vi "Area and Validity of a Triangle.vi"() -> ()   [LabVIEW 2011]
panel:
  out "Area of Triangle":dbl
  out "Valid Triangle?":bool
  in  "Side C (cm)":dbl=10.0
  in  "Side B (cm)":dbl=8.0
  in  "Side A (cm)":dbl=6.0
  # "Sides of a Triangle"
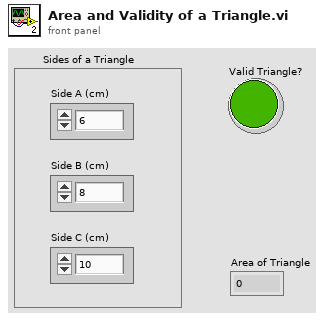
[diagram p1: front panel]
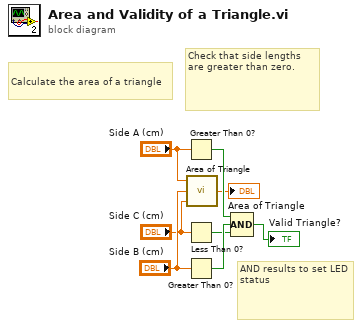
[diagram p0: block diagram]
diagram:
  # "AND results to set LED status"
  # "Check that side lengths are greater than zero."
  # "Calculate the area of a triangle"
  n1 = Greater Than 0?(x="Side A (cm)") -> (x > 0?=w8:bool)
  n2 = Less Than 0?(x="Side C (cm)") -> (x < 0?=w6:bool)
  n3 = Greater Than 0?(x="Side B (cm)") -> (x > 0?=w7:bool)
  n4 = call "Area of Triangle.vi"("Side C (cm)"="Side C (cm)", "Side B (cm)"="Side B (cm)", "Side A (cm)"="Side A (cm)") -> ("Area of Triangle (cm^2)"=→"Area of Triangle":dbl)
  n5 = Compound Arithmetic op=AND(w8, w7, w6) -> (→"Valid Triangle?":bool)
